vi "Config FX Set.vi"(5 "Max # Of Tries":i32, 6 "Send Cmd Timout(ms)":u32=300, 8 "Error":errorcluster, 9 "Grabber Config":T6={"Grabber Ver"=0, "CAN"={"ID"=0, "Bus"=""}, "Output"={"Type"=enum."Counter-Clockwise", "Neutral"=enum."EEPROMSetting", "Max"={"FWD"=0.0, "REV"=-1.0}, "Min"={"FWD"=0.0, "REV"=0.0}, "OL Ramp Rate (S)"=0.0, "Dead Band"=0.0}, "StatorLimit"={"Enable"=FALSE, "Current Limit"=0.0, "Threshold Current"=0.0, "Threshold Time"=0.0}} {"Output"."Min"."REV" format="%.2f"; "Output"."Min"."FWD" format="%.2f"; "Output"."Max"."REV" format="%.2f"; "Output"."Max"."FWD" format="%.2f"}, 11 "PhoenixMotorControlDevRef":T1={"DeviceStatus"={"status"=FALSE, "code"=0, "source"=""}, "Type"=enum."PWM", "PWM"={"PWM Channel"=enum."Invalid", "DeadBand"={"Name"="", "maxPositivePwm"=0, "minPositivePwm"=0, "centerPwm"=0, "maxNegativePwm"=0, "minNegativePwm"=0, "angularRange"=0}}, "CAN"={"Device Number"=0, "SetOutput VI Ref"=variant, "GetOutput VI Ref"=variant, "Enable VI Ref"=variant, "Disable VI Ref"=variant, "Data"=variant}, "Invert"=FALSE, "DIO PWM"={"PWM \"Enable\" Channel"=enum."Invalid", "DIOChannel"=enum."Invalid", "PWM Rate"=0.0}}) -> (0 "Error Out":errorcluster, 3 "PhoenixMotorControlDevRef Out Out":T1)   [LabVIEW 2020, in "Grabber_ACT.lvlib"]
uses:
  Grabber_ACT.lvlib
  <vilib>/Rock Robotics/WPI/MotorControl/WPI_MotorControlDeviceRef.ctl
  <vilib>/Rock Robotics/WPI/MotorControl/WPI_MotorControlType.ctl
  <vilib>/Rock Robotics/SystemInterfaces/DIO/FPGA_DIOPWMChannel.ctl
  <vilib>/Rock Robotics/WPI/PWM/WPI_PWMDeadband.ctl
  <vilib>/Rock Robotics/SystemInterfaces/DIO/FPGA_DIOChannel.ctl
  <vilib>/Utility/Data Type/NI_Data Type.lvlib
  <vilib>/Rock Robotics/WPI/ThirdParty/Phoenix-LabVIEW/Motor Controller/Controls/CTRE_Phoenix_MotorControl_NeutralMode.ctl
  <vilib>/Rock Robotics/WPI/ThirdParty/Phoenix-LabVIEW/Motor Controller/Controls/CTRE_Phoenix_MotorControl_TalonFXInvertType.ctl
  Shared Code/TypeDefs/Cluster_FWD  REV Values.ctl
  Shared Code/TypeDefs/Cluser_CAN Data.ctl
  Shared Code/TypeDefs/Cluster_Config Motor Output.ctl
  Shared Code/TypeDefs/Cluser_Config_Current Limits.ctl
  Shared Code/TypeDefs/Cluster_Grabber_Config FX Values.ctl
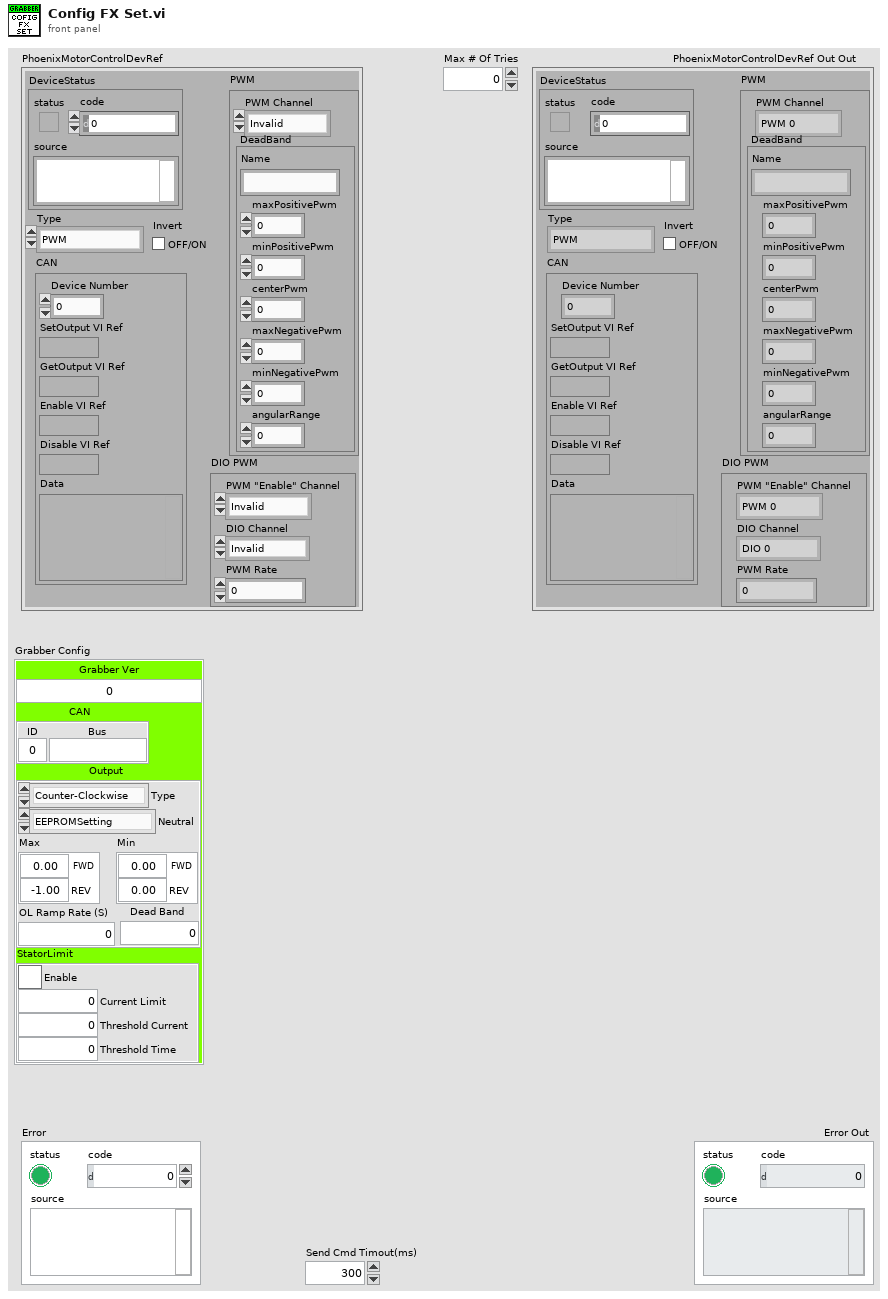
[diagram p1: front panel]
types:
  T1 = typedef "WPI_MotorControlDeviceRef.ctl" = cluster{"DeviceStatus":errorcluster, "Type":T2, "PWM":cluster{"PWM Channel":T3, "DeadBand":T4}, "CAN":cluster{"Device Number":u8, "SetOutput VI Ref":variant, "GetOutput VI Ref":variant, "Enable VI Ref":variant, "Disable VI Ref":variant, "Data":variant}, "Invert":bool, "DIO PWM":cluster{"PWM \"Enable\" Channel":T3, "DIOChannel":T5, "PWM Rate":dbl}}
  T2 = typedef "WPI_MotorControlType.ctl" = enum16{"PWM", "CAN", "DIO PWM"}
  T3 = typedef "FPGA_DIOPWMChannel.ctl" = enum8{"PWM 0", "PWM 1", "PWM 2", "PWM 3", "PWM 4", "PWM 5", "PWM 6", "PWM 7", "PWM 8", "PWM 9", "PWM MXP 0", "PWM MXP 1", "PWM MXP 2", "PWM MXP 3", "PWM MXP 4", "PWM MXP 5", "PWM MXP 6", "PWM MXP 7", "PWM MXP 8", "PWM MXP 9", "Invalid"}
  T4 = typedef "WPI_PWMDeadband.ctl" = cluster{"Name":string, "maxPositivePwm":i32, "minPositivePwm":i32, "centerPwm":i32, "maxNegativePwm":i32, "minNegativePwm":i32, "angularRange":u16}
  T5 = typedef "FPGA_DIOChannel.ctl" = enum8{"DIO 0", "DIO 1", "DIO 2", "DIO 3", "DIO 4", "DIO 5", "DIO 6", "DIO 7", "DIO 8", "DIO 9", "DIO MXP 0", "DIO MXP 1", "DIO MXP 2", "DIO MXP 3", "DIO MXP 4", "DIO MXP 5", "DIO MXP 6", "DIO MXP 7", "DIO MXP 8", "DIO MXP 9", "DIO MXP 10", "DIO MXP 11", "DIO MXP 12", "DIO MXP 13", "DIO MXP 14", "DIO MXP 15", "SPI Port CS1", "SPI Port CS2", "SPI Port CS3", "SPI Port MISO", "SPI Port MOSI", "Invalid"}
  T6 = typedef "Cluster_Grabber_Config FX Values.ctl" = cluster{"Grabber Ver":u64, "CAN":T7, "Output":T8, "StatorLimit":T12}
  T7 = typedef "Cluser_CAN Data.ctl" = cluster{"ID":u8, "Bus":string}
  T8 = typedef "Cluster_Config Motor Output.ctl" = cluster{"Type":T9, "Neutral":T10, "Max":T11, "Min":T11, "OL Ramp Rate (S)":dbl, "Dead Band":dbl}
  T9 = typedef "CTRE_Phoenix_MotorControl_TalonFXInvertType.ctl" = enum16{"Counter-Clockwise", "Clockwise"}
  T10 = typedef "CTRE_Phoenix_MotorControl_NeutralMode.ctl" = enum8{"EEPROMSetting", "Override to Coast", "Override to Brake"}
  T11 = typedef "Cluster_FWD  REV Values.ctl" = cluster{"FWD":dbl, "REV":dbl}
  T12 = typedef "Cluser_Config_Current Limits.ctl" = cluster{"Enable":bool, "Current Limit":dbl, "Threshold Current":dbl, "Threshold Time":dbl}
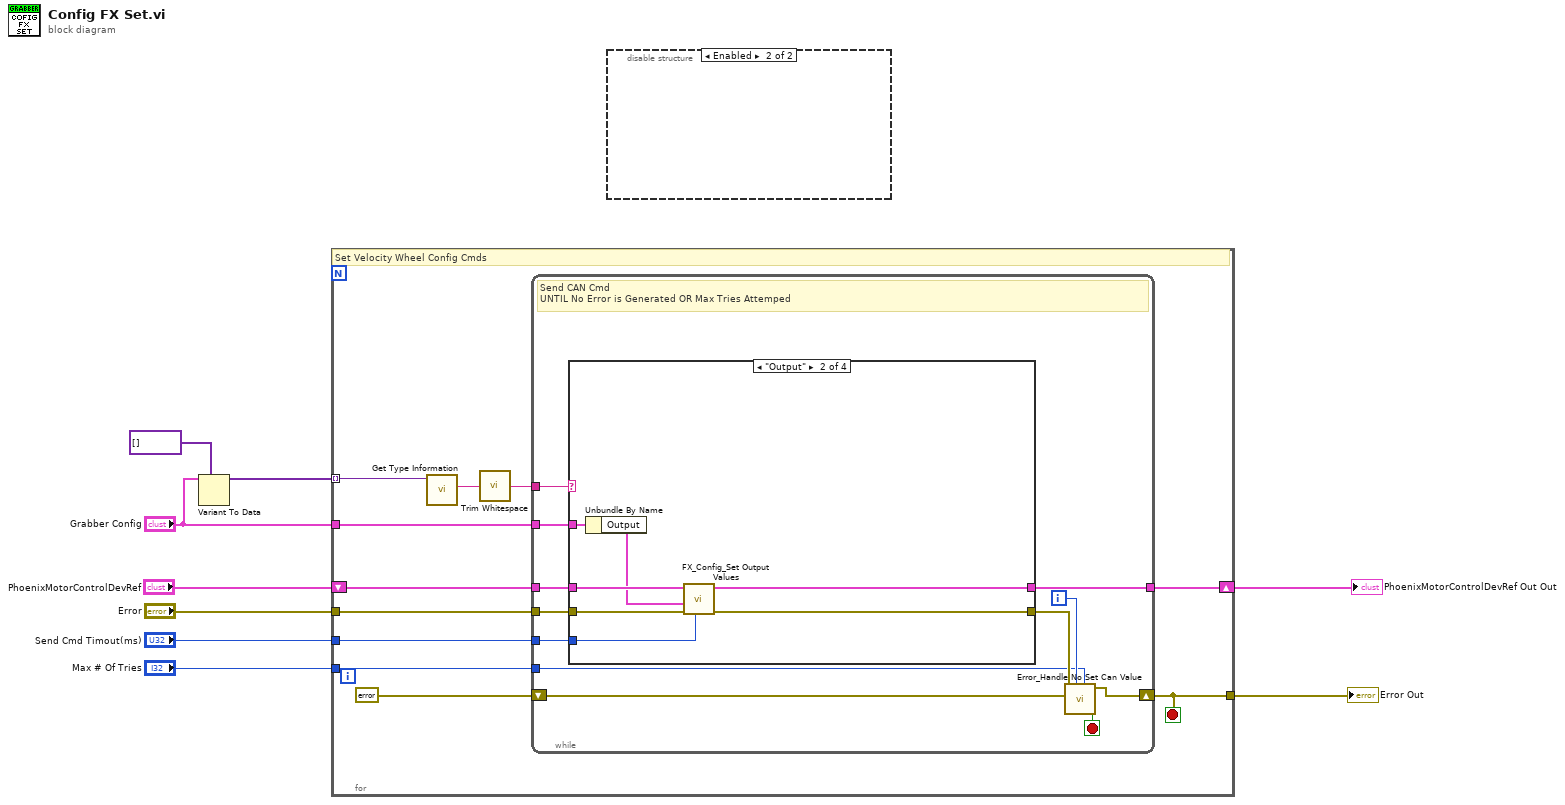
[diagram p0: block diagram]
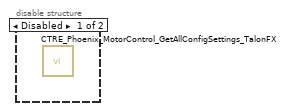
[diagram p2: hidden frame]
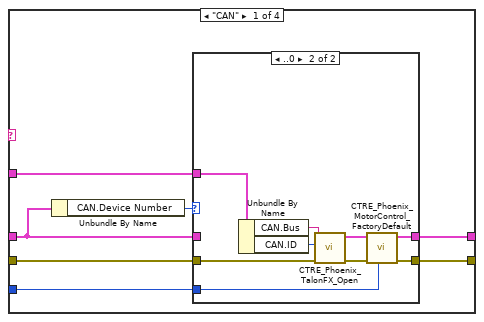
[diagram p3: hidden frame]
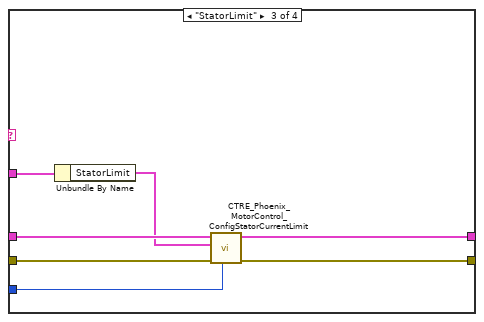
[diagram p5: hidden frame]
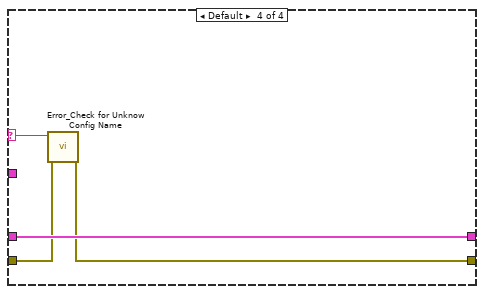
[diagram p6: hidden frame]
diagram:
  n1 = Variant To Data(type=variant[] [] ("appended array"), Variant="Grabber Config") -> (data=w1:variant[])  [unwired: 1 in, 1 out]
  n2 = for {
    tunnel: "Send Cmd Timout(ms)" -> [w19]
    shift-right: [w20] -> w6
    shift-left: "PhoenixMotorControlDevRef" -> [w17]
    tunnel: "Grabber Config" -> [w18]
    tunnel: "Max # Of Tries" -> [w15]
    tunnel: w1 -> [w14] mode=indexing
    tunnel: "Error" -> [w16]
    tunnel: [w13] -> w5
    stop <- w13 stop-if-true
    # "Set Velocity Wheel Config Cmds"
    n3 = call <vilib>:"Get Type Information.vi"("variant"=w14) -> ("name"=w11:string)  [unwired: 6 in, 4 out]
    n4 = call <vilib>:"Trim Whitespace.vi"("string"=w11) -> ("trimmed string"=w10:string)  [unwired: 1 in]
    n5 = while {
      tunnel: [w24] -> w20
      tunnel: w19 -> [w30]
      shift-right: [w31] -> w13
      shift-left: errorcluster {"status"=FALSE, "code"=0, "source"=""} ("Error Out") -> [w29]
      tunnel: w16 -> [w27]
      tunnel: w17 -> [w26]
      tunnel: w18 -> [w25]
      tunnel: w15 -> [w23]
      tunnel: w10 -> [w22]
      i -> [w28]
      stop <- w21 stop-if-true
      # "Send CAN Cmd\nUNTIL No Error is Generated OR Max Tries Attemped"
      n6 = case shown="\"Output\"" w22 {
        selector: w22 -> [_ _ _ w67]
        tunnel: [w39 w55 w61 w65] -> w32
        tunnel: w30 -> [w37 w53 w59 _]
        tunnel: w27 -> [w38 w54 w60 w66]
        tunnel: w26 -> [w35 w56 w62 w68]
        tunnel: w25 -> [w33 w52 w64 _]
        tunnel: [w34 w57 w63 w68] -> w24
        frame "CAN" {
          n7 = Unbundle By Name(w35) -> ("CAN.Device Number"=w36:u8)
          n8 = case shown="..0" w36 {
            tunnel: [w40 w47] -> w39
            tunnel: w38 -> [w40 w46]
            tunnel: w37 -> [_ w45]
            tunnel: w35 -> [w41 _]
            tunnel: [w41 w43] -> w34
            tunnel: w33 -> [_ w42]
            frame 1.. {
            }
            frame ..0 {
              n9 = Unbundle By Name(w42) -> ("CAN.Bus"=w44:string, "CAN.ID"=w48:u8)
              n10 = call <vilib>:"CTRE_Phoenix_TalonFX_Open.vi"("error in"=w46, "Device Number"=w48, "CAN Bus"=w44) -> ("error out"=w49:errorcluster, "PhoenixMotorControlDevRef"=w50:T1)  [unwired: 7 in]
              n11 = call <vilib>:"CTRE_Phoenix_MotorControl_FactoryDefault.vi"("timeoutMs"=w45, "error in"=w49, "PhoenixMotorControlDevRef"=w50) -> ("error out"=w47:errorcluster, "PhoenixMotorControlDevRef"=w43:T1)  [unwired: 7 in]
            }
          }
        }
        frame "Output" {
          n12 = Unbundle By Name(w52) -> ("Output"=w51:T8)
          n13 = call "FX_Config_Set Output Values.vi"("Send Cmd Timout(ms)"=w53, "Error"=w54, "Output"=w51, "PhoenixMotorControlDevRef"=w56) -> ("Error Out"=w55:errorcluster, "PhoenixMotorControlDevRef Out"=w57:T1)  [unwired: 6 in]
        }
        frame "StatorLimit" {
          n14 = Unbundle By Name(w64) -> ("StatorLimit"=w58:T12)
          n15 = call <vilib>:"CTRE_Phoenix_MotorControl_ConfigStatorCurrentLimit.vi"("timeoutMs"=w59, "error in (no error)"=w60, "Stator Current Limit Configuration"=w58, "PhoenixMotorControlDevRef"=w62) -> ("error out"=w61:errorcluster, "PhoenixMotorControlDevRef"=w63:T1)  [unwired: 6 in]
        }
        frame Default {
          n16 = call "Error_Check for Unknow Config Name.vi"("error in (no error)"=w66, "Config Name"=w67) -> ("error out"=w65:errorcluster)  [unwired: 9 in]
        }
      }
      n17 = call "Error_Handle No Set Can Value.vi"("Max # Of Tries"=w23, "Loop Itteration"=w28, "Previous Error"=w29, "Error"=w32) -> ("Stop Out"=w21:bool, "Error Out"=w31:errorcluster)  [unwired: 6 in]
    }
  }
  "Error Out" <- w5
  "PhoenixMotorControlDevRef Out Out" <- w6
  n18 = disable-structure shown="Enabled" {
    frame Disabled {
      n19 = call <vilib>:"CTRE_Phoenix_MotorControl_GetAllConfigSettings_TalonFX.vi"() -> ()  [unwired: 9 in, 3 out]
    }
    frame Enabled {
    }
  }
